vi "test_Write Cluster Register Value.vi"(8 "error in (no error)":errorcluster, 11 "TestCase in":refnum<class "FPGA Register IO Tests.lvclass">) -> (0 "error out":errorcluster, 3 "TestCase out":refnum<class "FPGA Register IO Tests.lvclass">)   [LabVIEW 2021, in "FPGA Register IO Tests.lvclass"]
uses:
  FPGA Register IO Tests.lvclass
  FPGA Register IO Tests.lvclass/FPGA Register IO Tests.ctl
  ac679e79-fbfa-4f1c-b8b2-6e0ee038be99.vi
  7771d823-460b-4368-a3f4-a2f2703818a4.vi
  APIs/FPGA Register IO/SubVIs/Parse Cluster Configuration.vi
  APIs/FPGA Register IO/Write Methods/Write Data Register/Instances/Write U8 Array.vi
  APIs/FPGA Register IO/Read Methods/Read Data Register/Instances/Read U8 Array.vi
  APIs/FPGA Register IO/SubVIs/Check Cluster Configuration Store.vi
  APIs/FPGA Register IO/Utilities/Find Register Offset.vi
  APIs/FPGA Register IO/SubVIs/Check Register Data Store.vi
  <userlib>/_OpenG.lib/lvdata/lvdata.llb/Variant to Header Info__ogtk.vi
  <userlib>/_OpenG.lib/lvdata/lvdata.llb/Split Cluster TD__ogtk.vi
  <userlib>/_OpenG.lib/lvdata/lvdata.llb/Cluster to Array of VData__ogtk.vi
  <vilib>/Utility/Data Type/Get Type Information.vi
  <userlib>/_OpenG.lib/lvdata/lvdata.llb/Get Strings from Enum__ogtk.vi
  APIs/FPGA Register IO/Error Handling/Error 6004.vi
  <vilib>/Utility/Data Type/Get Fixed-Point Information.vi
  APIs/FPGA Register IO/Error Handling/Error 6001.vi
  APIs/FPGA Register IO/Error Handling/Error 6000.vi
  APIs/FPGA Register IO/Error Handling/Error 6002.vi
  APIs/FPGA Register IO/Error Handling/Error 6006.vi
  APIs/FPGA Register IO/Error Handling/Error 6003.vi
  <vilib>/FPGAPlugInAG/Dynamic/niLvFpga_Close_Dynamic.vi
  <vilib>/rvi/interface/nirviCloseFPGA/nirviCloseFPGA.xnode
  <vilib>/addons/_JKI Toolkits/VI Tester/TestCase.llb/TestCase.lvclass
  APIs/FPGA Register IO/FPGA Register IO.lvlib
  C:/Program Files/National Instruments/LabVIEW 2021/vi.lib/addons/_JKI Toolkits/VI Tester/TestCase.llb/TestCase.lvclass
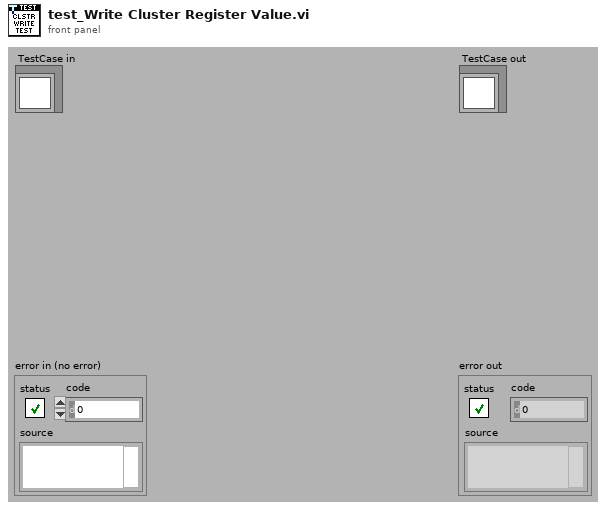
[diagram p1: front panel]
types:
  T1 = cluster{"I16":i16, "U64":u64, "SGL":sgl, "Bool":bool, "FXP 12/6":fxp<+/-,12,6>}
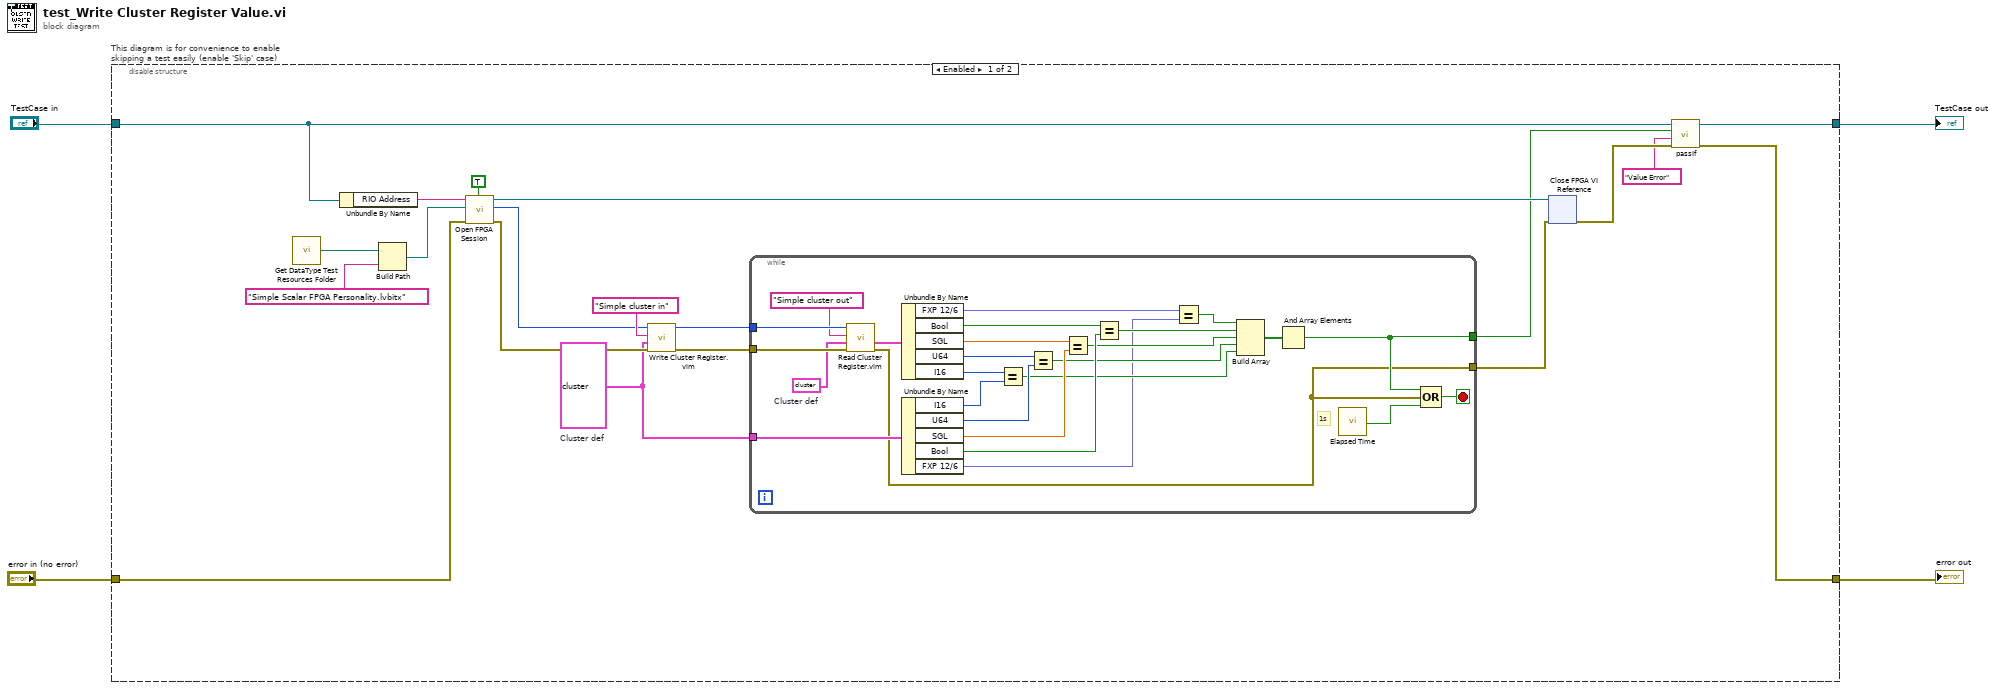
[diagram p0: block diagram]
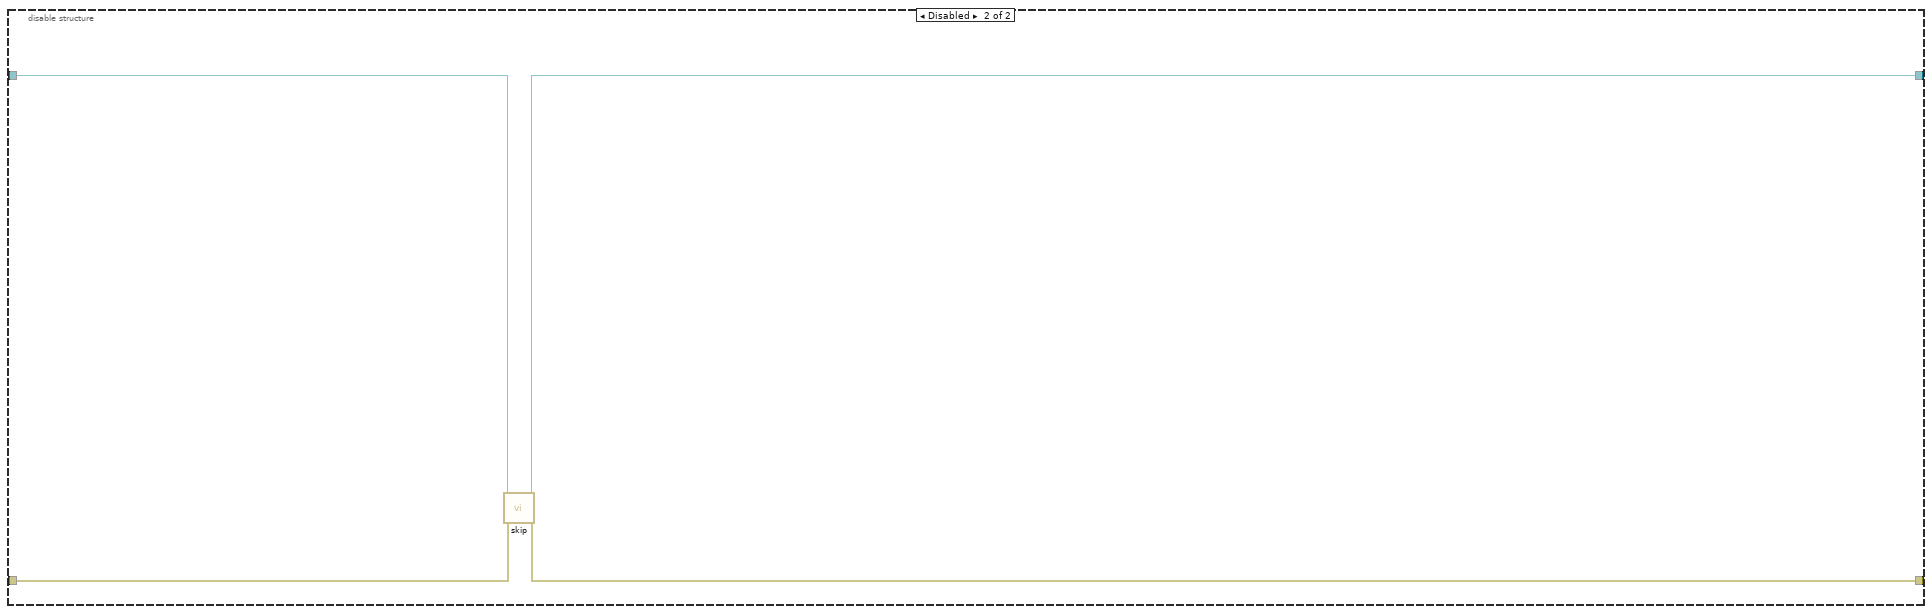
[diagram p2: hidden frame]
diagram:
  n1 = disable-structure "This diagram is for convenience to enable skipping a test easily (enable 'Skip' case)" shown="Enabled" {
    disable-tunnel: "TestCase in" -> [w18 w54]
    disable-tunnel: [w13 w52] -> w1
    disable-tunnel: [w14 w53] -> w3
    disable-tunnel: "error in (no error)" -> [w19 w51]
    frame Enabled {
      w7 = T1 {"I16"=10, "U64"=100, "SGL"=9.0, "Bool"=TRUE, "FXP 12/6"=1.09375}  # Cluster def
      n2 = call "Get DataType Test Resources Folder.vi"() -> ("path"=w16:path)
      n3 = Unbundle By Name(w18) -> ("RIO Address"=w21:string)
      n4 = Build Path(base path=w16, name or relative path="Simple Scalar FPGA Personality.lvbitx") -> (appended path=w20:path)
      n5 = call "Open FPGA Session.vi"("run when loaded (T)"=TRUE ("Run When Loaded (T)"), "error in"=w19, "bitfile path"=w20, "device address"=w21) -> ("error out"=w12:errorcluster, "session out"=w10:u32, "bitfile reference out"=w23:refnum<k20>)  [unwired: 5 in]
      n6 = call "Write Cluster Register.vim"("error in (no error)"=w12, "Cluster in"=w7, "Cluster Name"="Simple cluster in" ("registerName"), "session in"=w10) -> ("error out"=w8:errorcluster, "session out"=w9:u32)  [unwired: 6 in]
      n7 = while {
        tunnel: w8 -> [w48]
        tunnel: w9 -> [w47]
        tunnel: [w29] -> w6
        tunnel: w7 -> [w44]
        tunnel: [w28] -> w5
        stop <- w50 stop-if-true
        w27 = T1 {"I16"=0, "U64"=0, "SGL"=0.0, "Bool"=FALSE, "FXP 12/6"=0.0}  # Cluster def
        # "1s"
        n8 = call "Read Cluster Register.vim"("error in (no error)"=w48, "Cluster in (default value)"=w27, "Cluster Name"="Simple cluster out" ("registerName"), "session in"=w47) -> ("error out"=w28:errorcluster, "Cluster out"=w45:T1)  [unwired: 4 in, 2 out]
        n9 = Unbundle By Name(w45) -> ("FXP 12/6"=w26:fxp<+/-,12,6>, "Bool"=w37:bool, "SGL"=w39:sgl, "U64"=w40:u64, "I16"=w42:i16)
        n10 = Unbundle By Name(w44) -> ("I16"=w43:i16, "U64"=w41:u64, "SGL"=w38:sgl, "Bool"=w36:bool, "FXP 12/6"=w25:fxp<+/-,12,6>)
        n11 = Equal?(x=w42, y=w43) -> (x = y?=w31:bool)
        n12 = Equal?(x=w40, y=w41) -> (x = y?=w32:bool)
        n13 = Equal?(x=w39, y=w38) -> (x = y?=w33:bool)
        n14 = Equal?(x=w37, y=w36) -> (x = y?=w34:bool)
        n15 = Equal?(x=w26, y=w25) -> (x = y?=w35:bool)
        n16 = Build Array(w35, w34, w33, w32, w31) -> (w30:bool[])
        n17 = And Array Elements(Boolean array=w30) -> (logical AND=w29:bool)
        n18 = call "Elapsed Time"() -> ("Time has Elapsed"=w49:bool)  [unwired: 12 in, 7 out]
        n19 = Compound Arithmetic op=OR(w29, w28, w49) -> (w50:bool)
      }
      n20 = xnode "Close FPGA VI Reference"("FPGA VI Reference In"=w23, "error in"=w5) -> ("error out"=w17:errorcluster)
      n21 = call-dynamic "passIf.vi"("error in (no error)"=w17, "message (\"\")"="Value Error" ("message (\"\")"), "pass"=w6, "TestCase in"=w18) -> ("error out"=w14:errorcluster, "TestCase out"=w13:refnum<class "FPGA Register IO Tests.lvclass">)  [unwired: 6 in]
    }
    frame Disabled {
      # "skip test result while test is under development"
      n22 = call <vilib>:"skip.vi"("error in (no error)"=w51, "TestCase in"=w54) -> ("error out"=w53:errorcluster, "TestCase out"=w52:refnum<class "FPGA Register IO Tests.lvclass">)  [unwired: 8 in]
    }
  }
  "error out" <- w3
  "TestCase out" <- w1
